vi "read_test.vi"(8 "错误输入（无错误）":errorcluster, 10 "基地址":u32=1048576 format="%.0x", 11 "VISA资源名称":refnum<visa-resource-name>) -> (0 "错误输出":errorcluster, 2 "U8":u8[](array[numeric]), 3 "VISA资源名称输出":refnum<visa-resource-name>)   [LabVIEW 2012]
uses:
  <vilib>/Instr/_visa.llb/VISA Register Access Address Space.ctl
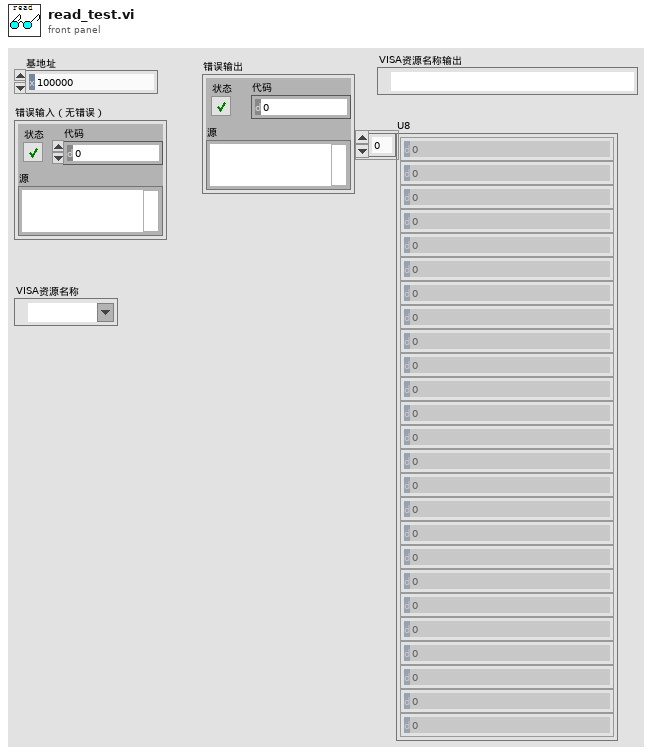
[diagram p1: front panel]
types:
  T1 = typedef "VISA Register Access Address Space.ctl" = u16
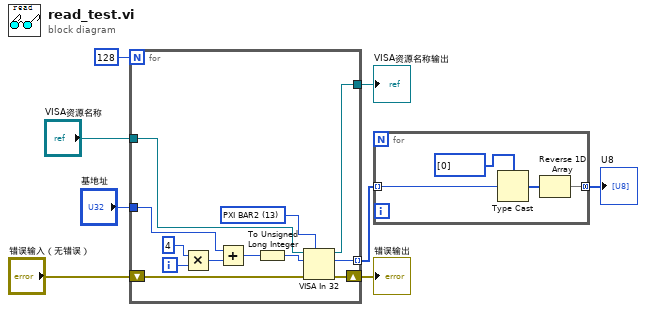
[diagram p0: block diagram]
diagram:
  n1 = for {
    N: 128 -> [_]
    tunnel: "基地址" -> [w17]
    tunnel: [w16] -> w1 mode=indexing
    tunnel: "VISA资源名称" -> [w15]
    shift-right: [w12] -> w4
    shift-left: "错误输入（无错误）" -> [w13]
    tunnel: [w11] -> w2
    i -> [w19]
    w14 = T1 13 items=["VXI/VME A16"=1, "VXI/VME A24"=2, "VXI/VME A32"=3, "VXI/VME A64"=4, "PXI内存分配"=9, "PXI配置"=10, "PXI BAR0"=11, "PXI BAR1"=12, "PXI BAR2"=13, "PXI BAR3"=14, "PXI BAR4"=15, "PXI BAR5"=16] ("Address Space")
    n2 = Multiply(x=4, y=w19) -> (x*y=w20:i32)
    n3 = Add(x=w17, y=w20) -> (x+y=w10:u32)
    n4 = To Unsigned Long Integer(number=w10) -> (unsigned 32bit integer=w9:u32)
    n5 = VISA In 32(7:w14, 8:w13, 10:w9, 11:w15) -> (0:w12:errorcluster, 2:w16:u32, 3:w11:refnum<visa-resource-name>)
  }
  "错误输出" <- w4
  "VISA资源名称输出" <- w2
  n6 = for {
    tunnel: [w21] -> w3 mode=concatenating
    tunnel: w1 -> [w22] mode=indexing
    n7 = Type Cast(type=u8[] [0], x=w22) -> (*(type *) &x=w23:u8[])
    n8 = Reverse 1D Array(array=w23) -> (reversed array=w21:u8[])
  }
  "U8" <- w3
